vi "DAQmx.Create.vi"(8 "error in":errorcluster, 11 "DAQmx in":refnum<class "DAQmx.lvclass">) -> (0 "error out":errorcluster, 3 "DAQmx out":refnum<class "DAQmx.lvclass">)   [LabVIEW 2019, in "DAQmx.lvclass"]
uses:
  DAQmx.lvclass
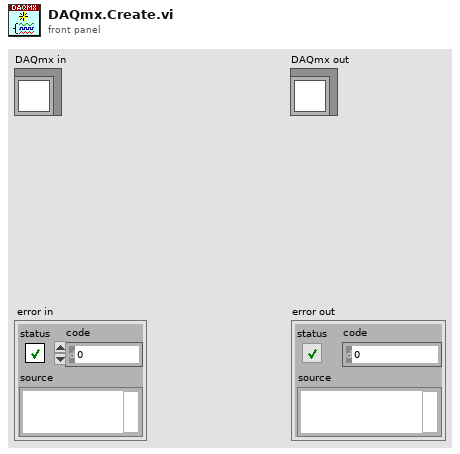
[diagram p1: front panel]
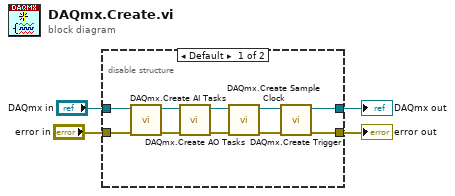
[diagram p0: block diagram]
diagram:
  n1 = disable-structure shown="Default" {
    disable-tunnel: "DAQmx in" -> [w8 w16]
    disable-tunnel: "error in" -> [w7 w15]
    disable-tunnel: [w10 w16] -> w3
    disable-tunnel: [w9 w15] -> w2
    frame condition #0 (active) {
      n2 = call "DAQmx.Create AI Tasks.vi"("error in"=w7, "DAQmx in"=w8) -> ("error out"=w11:errorcluster, "DAQmx out"=w12:refnum<class "DAQmx.lvclass">)  [unwired: 8 in]
      n3 = call "DAQmx.Create AO Tasks.vi"("error in (no error)"=w11, "DAQmx in"=w12) -> ("error out"=w13:errorcluster, "DAQmx out"=w14:refnum<class "DAQmx.lvclass">)  [unwired: 8 in]
      n4 = call "DAQmx.Create Sample Clock.vi"("error in (no error)"=w13, "DAQmx in"=w14) -> ("error out"=w5:errorcluster, "DAQmx out"=w6:refnum<class "DAQmx.lvclass">)  [unwired: 8 in]
      n5 = call "DAQmx.Create Trigger.vi"("error in (no error)"=w5, "DAQmx in"=w6) -> ("error out"=w9:errorcluster, "DAQmx out"=w10:refnum<class "DAQmx.lvclass">)  [unwired: 8 in]
    }
    frame condition #1 {
    }
  }
  "error out" <- w2
  "DAQmx out" <- w3
